vi "Get Builder Cluster.vi"(8 "error in (no error)":errorcluster, 10 "VI Refnum":refnum<vi>, 11 "Panel Form Controller in":refnum<class "Panel Form Controller.lvclass">) -> (0 "error out":errorcluster, 2 "Builder Cluster":T1, 3 "Panel Form Controller out":refnum<class "Panel Form Controller.lvclass">)   [LabVIEW 2020, in "Panel Form Controller.lvlib" / "Panel Form Controller.lvclass"]
uses:
  Panel Form Controller.lvclass
  Builder Cluster.ctl
  Field.lvclass
  Button.lvclass
  Panel Form Controller.lvclass/Panel Form Controller.ctl
  Field.lvclass/Field.ctl
  Panel Form Controller.lvlib
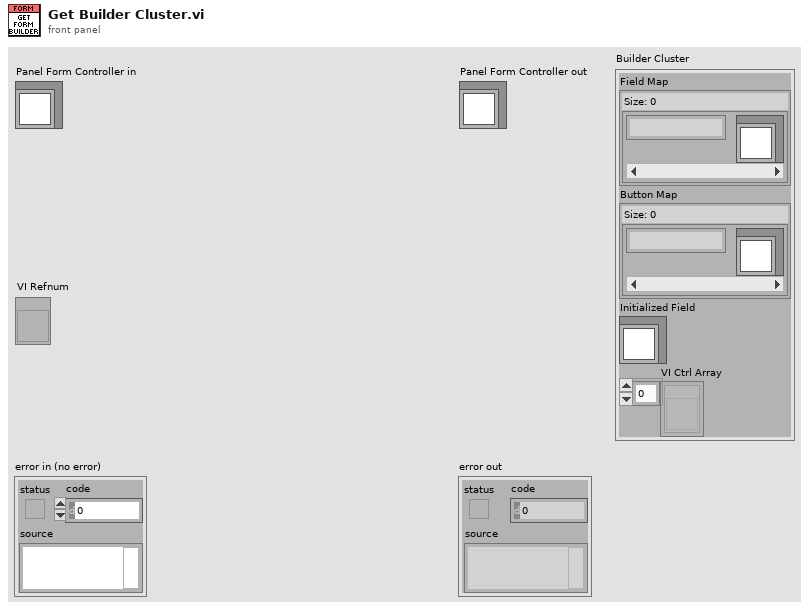
[diagram p1: front panel]
types:
  T1 = typedef "Panel Form Controller.lvlib/Builder Cluster.ctl" = cluster{"Field Map":map{string, refnum<class "Field.lvclass">}, "Button Map":map{string, refnum<class "Button.lvclass">}, "Initialized Field":refnum<class "Field.lvclass">, "VI Ctrl Array":refnum<vi>[]}
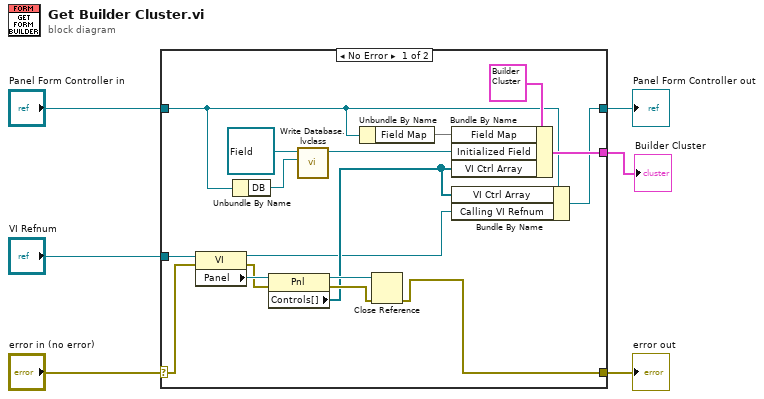
[diagram p0: block diagram]
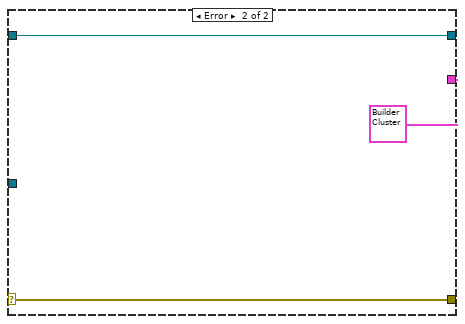
[diagram p2: hidden frame]
diagram:
  n1 = case shown="No Error" "error in (no error)" {
    selector: "error in (no error)" -> [w13 w26]
    tunnel: [w7 w26] -> w5
    tunnel: [w10 w25] -> w3
    tunnel: "Panel Form Controller in" -> [w11 w25]
    tunnel: "VI Refnum" -> [w21 _]
    tunnel: [w12 T1 {"Field Map"={}, "Button Map"={}, "Initialized Field"=refnum, "VI Ctrl Array"=[]} ("Builder Cluster")] -> w1
    frame No Error {
      n2 = property class="VI"(reference=w21, error in=w13) -> (reference out=w8:refnum<vi>, error out=w19:errorcluster, "Panel"=w20:refnum<vi>)
      n3 = Unbundle By Name(w11) -> ("DB"=w22:refnum<class "Database.lvclass">)
      n4 = property class="Pnl"(reference=w20, error in=w19) -> (reference out=w15:refnum<vi>, error out=w14:errorcluster, "Controls[]"=w9:refnum<vi>[])
      n5 = call "Write Database.lvclass.vi"("Database.lvclass"=w22, "Field in"=refnum<class "Field.lvclass"> refnum ("Field.lvclass")) -> ("Field out"=w17:refnum<class "Field.lvclass">)  [unwired: 8 in, 1 out]
      n6 = Unbundle By Name(w11) -> ("Field Map"=w16:map{string, refnum<class "Field.lvclass">})
      n7 = Close Reference(reference=w15, error in (no error)=w14) -> (error out=w7:errorcluster)
      n8 = Bundle By Name(cluster=T1 {"Field Map"={}, "Button Map"={}, "Initialized Field"=refnum, "VI Ctrl Array"=[]} ("Builder Cluster"), "Field Map"=w16, "Initialized Field"=w17, "VI Ctrl Array"=w9) -> (w12:T1)
      n9 = Bundle By Name(cluster=w11, "VI Ctrl Array"=w9, "Calling VI Refnum"=w8) -> (w10:refnum<class "Panel Form Controller.lvclass">)
    }
    frame Error {
    }
  }
  "error out" <- w5
  "Panel Form Controller out" <- w3
  "Builder Cluster" <- w1
